vi "PulseParseRF.vi"(0 "String":string) -> (2 "Array":variant[](array[variant]))   [LabVIEW 2017]
panel:
  out "output cluster":T1
  in  "Channel cluster":T2(array[cluster])
  in  "Timing cluster":T3
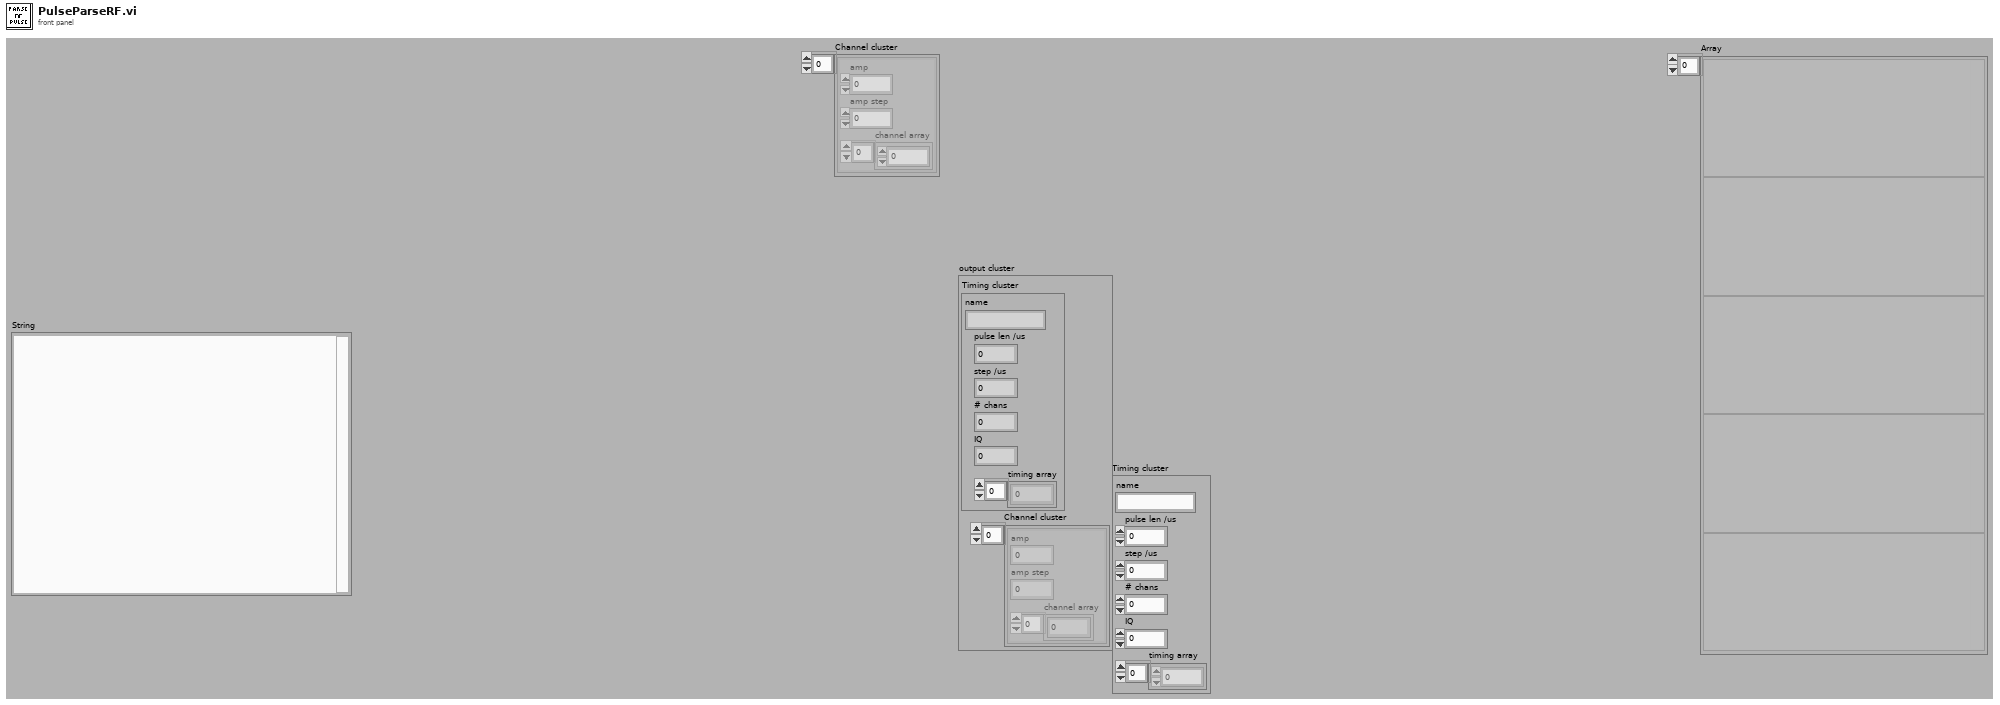
[diagram p1: front panel]
types:
  T1 = cluster{"Timing cluster":cluster{"name":string, "pulse len /us":dbl, "step /us":dbl, "# chans":i32, "IQ":i32, "timing array":dbl[]}, "Channel cluster":cluster{"amp":dbl, "amp step":dbl, "channel array":dbl[]}[]}
  T2 = cluster{"amp":dbl, "amp step":dbl, "channel array":dbl[]}[]
  T3 = cluster{"name":string, "pulse len /us":dbl, "step /us":dbl, "# chans":i32, "IQ":i32, "timing array":dbl[]}
  T4 = cluster{"Timing cluster 2":cluster{"name":string, "pulse len /us":dbl, "step /us":dbl, "# chans":i32, "IQ":i32, "timing array":dbl[]}, "Channel cluster 2":cluster{"amp":dbl, "amp step":dbl, "channel array":dbl[]}[]}
  T5 = cluster{"amp":dbl, "amp step":dbl, "array type (2D Dbl)":dbl[]}
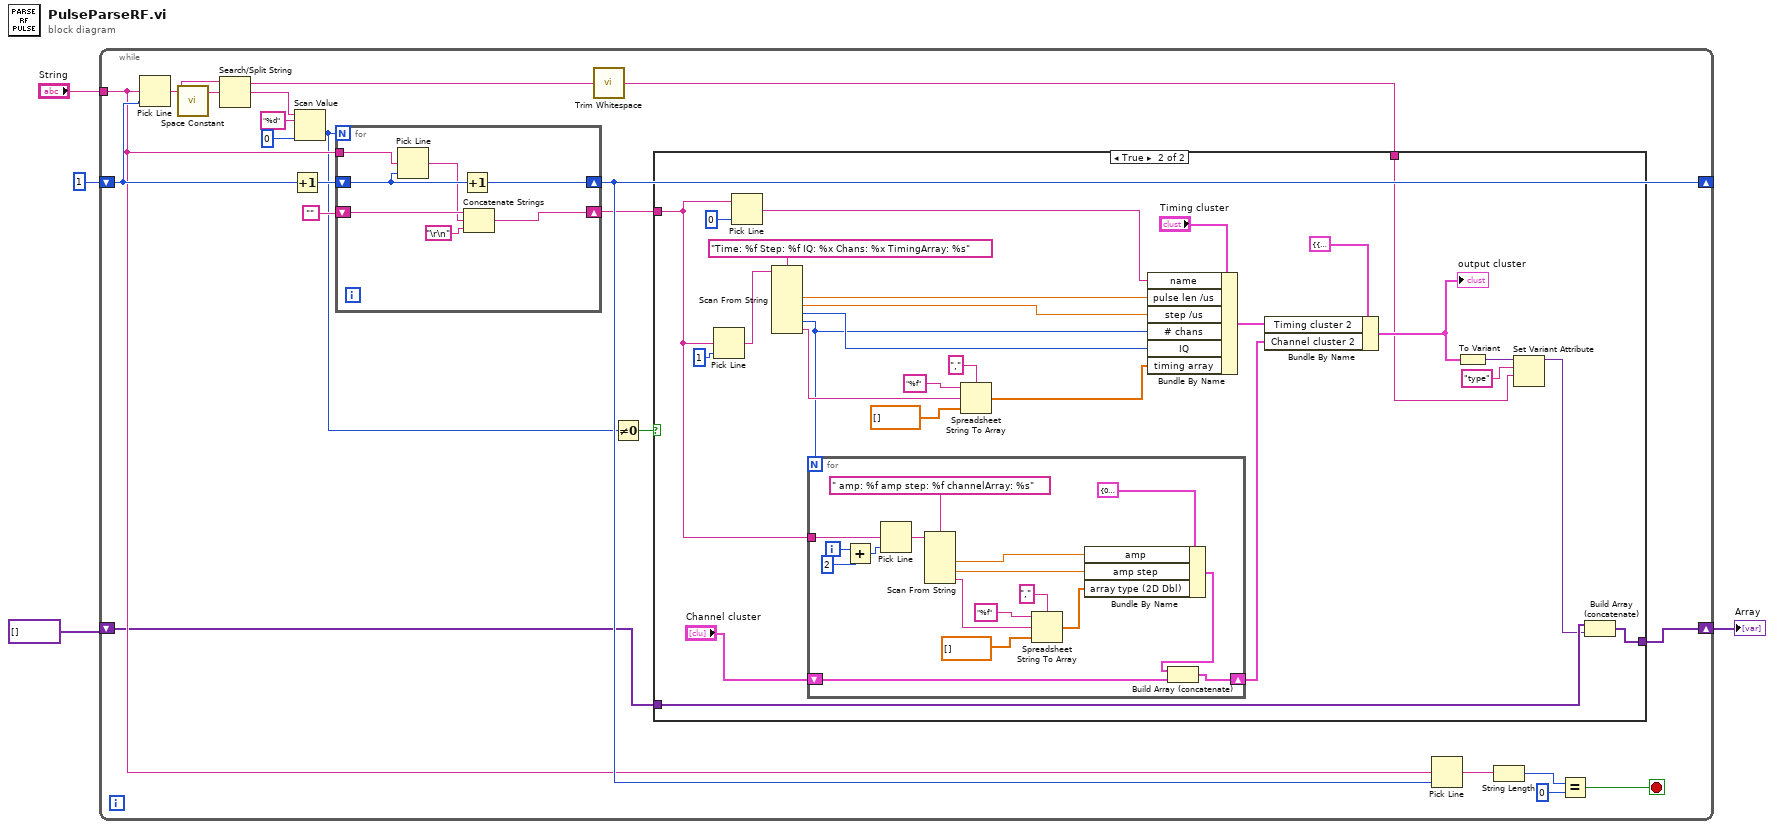
[diagram p0: block diagram]
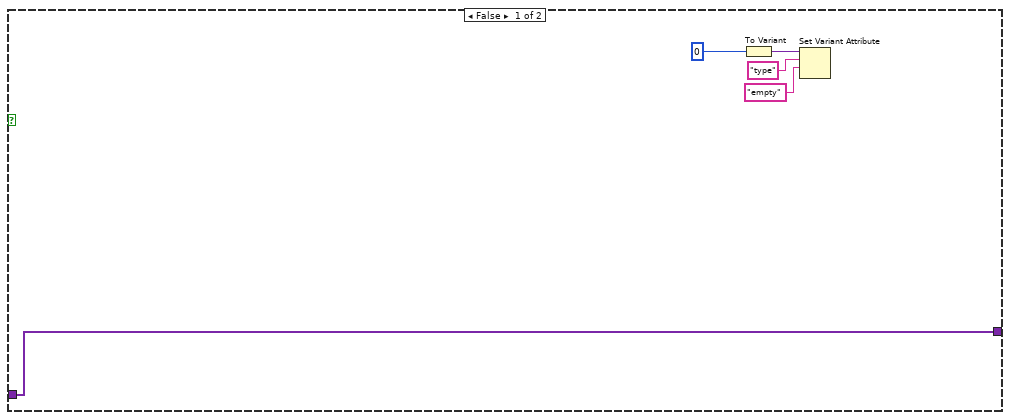
[diagram p2: hidden frame]
diagram:
  n1 = while {
    tunnel: "String" -> [w12]
    shift-right: [w13] -> _
    shift-left: 1 -> [w19]
    shift-right: [w6] -> w1
    shift-left: variant[] [] -> [w5]
    stop <- w14 stop-if-true
    n2 = Pick Line(multi-line string=w12, line index=w19) -> (output string=w25:string)  [unwired: 1 in]
    n3 = call <vilib>:"Space Constant.vi"() -> ("String"=w24:string)
    n4 = Search/Split String(string=w25, search string/char (-)=w24) -> (substring before match=w23:string, match + rest of string=w22:string)  [unwired: 1 in, 1 out]
    n5 = Increment(x=w19) -> (x+1=w18:i32)
    n6 = Scan Value(string=w22, format string="%d", default (0 dbl)=0) -> (value=w7:i32)  [unwired: 1 out]
    n7 = for {
      N: w7 -> [_]
      tunnel: w12 -> [w79]
      shift-right: [w81] -> w13
      shift-left: w18 -> [w80]
      shift-right: [w75] -> w11
      shift-left: "" -> [w78]
      n8 = Pick Line(multi-line string=w79, line index=w80) -> (output string=w77:string)  [unwired: 1 in]
      n9 = Increment(x=w80) -> (x+1=w81:i32)
      n10 = Concatenate Strings(w78, w77, "\r\n") -> (w75:string)
    }
    n11 = call <vilib>:"Trim Whitespace.vi"("string"=w23) -> ("trimmed string"=w9:string)  [unwired: 1 in]
    n12 = Not Equal To 0?(x=w7) -> (x != 0?=w8:bool)
    n13 = case shown="True" w8 {
      tunnel: w11 -> [_ w57]
      tunnel: w9 -> [_ w35]
      tunnel: [w26 w33] -> w6
      tunnel: w5 -> [w26 w32]
      frame False {
        n14 = To Variant(anything=0) -> (Variant=w29:variant)
        n15 = Set Variant Attribute(Variant=w29, name="type", value="empty" ("name")) -> ()  [unwired: 1 in, 3 out]
      }
      frame True {
        n16 = Pick Line(multi-line string=w57, line index=1) -> (output string=w56:string)  [unwired: 1 in]
        n17 = Pick Line(multi-line string=w57, line index=0) -> (output string=w42:string)  [unwired: 1 in]
        n18 = Scan From String(format string="Time: %f Step: %f IQ: %x Chans: %x TimingArray: %s", input string=w56) -> (output 1=w54:dbl, output 2=w55:dbl, output 3=w45:u32, output 4=w44:u32, output 5=w47:string)  [unwired: 7 in, 3 out]
        n19 = for {
          N: w44 -> [_]
          shift-right: [w62] -> w39
          shift-left: "Channel cluster" -> [w63]
          tunnel: w57 -> [w73]
          i -> [w72]
          n20 = Add(x=w72, y=2) -> (x+y=w71:i32)
          n21 = Pick Line(multi-line string=w73, line index=w71) -> (output string=w69:string)  [unwired: 1 in]
          n22 = Scan From String(format string=" amp: %f amp step: %f channelArray: %s", input string=w69) -> (output 1=w58:dbl, output 2=w59:dbl, output 3=w65:string)  [unwired: 5 in, 3 out]
          n23 = Spreadsheet String To Array(delimiter (Tab)=",", format string="%f", spreadsheet string=w65, array type (2D Dbl)=dbl[] []) -> (array=w60:dbl[])
          n24 = Bundle By Name(cluster=T5 {"amp"=0.0, "amp step"=0.0, "array type (2D Dbl)"=[]} ("freq cluster"), "amp"=w58, "amp step"=w59, "array type (2D Dbl)"=w60) -> (w61:T5)
          n25 = Build Array (concatenate)(w61, w63) -> (w62:T2)
        }
        n26 = Spreadsheet String To Array(delimiter (Tab)=",", format string="%f", spreadsheet string=w47, array type (2D Dbl)=dbl[] []) -> (array=w43:dbl[])
        n27 = Bundle By Name(cluster="Timing cluster", "name"=w42, "pulse len /us"=w54, "step /us"=w55, "# chans"=w44, "IQ"=w45, "timing array"=w43) -> (w40:T3)
        n28 = Bundle By Name(cluster=T4 {"Timing cluster 2"={"name"="", "pulse len /us"=0.0, "step /us"=0.0, "# chans"=0, "IQ"=0, "timing array"=[]}, "Channel cluster 2"=[]} ("RF pulse cluster"), "Timing cluster 2"=w40, "Channel cluster 2"=w39) -> (w38:T4)
        "output cluster" <- w38
        n29 = To Variant(anything=w38) -> (Variant=w37:variant)
        n30 = Set Variant Attribute(Variant=w37, name="type", value=w35) -> (Variant out=w31:variant)  [unwired: 1 in, 2 out]
        n31 = Build Array (concatenate)(w32, w31) -> (w33:variant[])
      }
    }
    n32 = Pick Line(multi-line string=w12, line index=w13) -> (output string=w17:string)  [unwired: 1 in]
    n33 = String Length(string=w17) -> (length=w16:i32)
    n34 = Equal?(x=w16, y=0) -> (x = y?=w14:bool)
  }
  "Array" <- w1
